vi "error log fg.vi"(2 "Error":string, 3 "Log Mode":enum16{"Get", "Set", "Clear"}(ring)) -> (0 "Errors":string, 1 "Errors Present":bool)   [LabVIEW 2013]
panel:
  # "Error Logging FG"
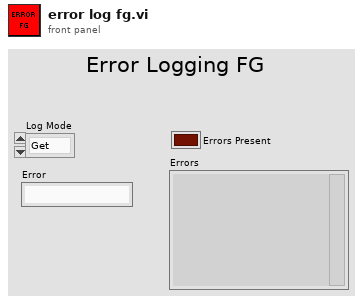
[diagram p1: front panel]
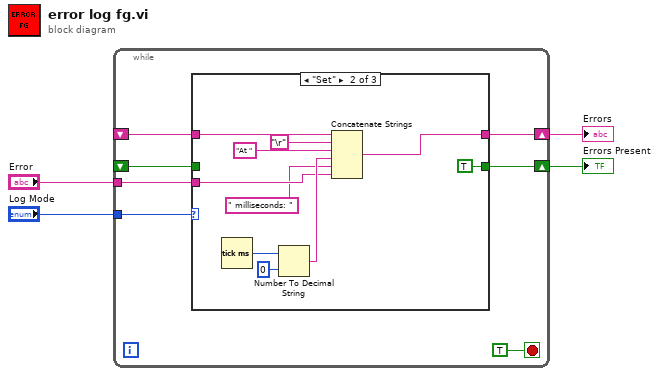
[diagram p0: block diagram]
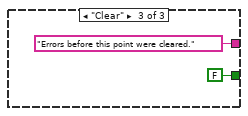
[diagram p3: hidden frame]
diagram:
  n1 = while {
    tunnel: "Error" -> [w9]
    shift-right: [w10] -> w2
    shift-left: _ -> [w8]
    tunnel: "Log Mode" -> [w11]
    shift-right: [w6] -> w1
    shift-left: _ -> [w5]
    stop <- TRUE stop-if-true
    n2 = case shown="\"Set\"" w11 {
      tunnel: [w13 w23 "Errors before this point were cleared."] -> w10
      tunnel: w9 -> [_ w15 _]
      tunnel: w8 -> [w13 w22 _]
      tunnel: [w12 TRUE FALSE] -> w6
      tunnel: w5 -> [w12 _ _]
      frame "Get", Default {
      }
      frame "Set" {
        n3 = Tick Count (ms)() -> (millisecond timer value=w19:u32)
        n4 = Number To Decimal String(number=w19, width (-)=i16 0) -> (decimal integer string=w16:string)
        n5 = Concatenate Strings(w22, "\r", "At ", w16, " milliseconds: ", w15) -> (w23:string)
      }
      frame "Clear" {
      }
    }
  }
  "Errors" <- w2
  "Errors Present" <- w1
